vi "OAT Torsional Vibration (Analog Tacho) (Even-Angle) (N Ch - 1 Setting).vi"(0 "analog tacho signals":waveform(dbl)[](array[waveform]), 1 "threshold (auto)":dbl=inf, 2 "pulse/revolution (1)":i32=1 min=1, 3 "hysteresis (0)":dbl format="%.2g", 4 "torsional vibration units":enum16{"RPM", "deg/s", "rad/s"}(ring), 5 "error in (no error)":errorcluster, 6 "missing pulses? (no:F)":bool, 7 "pulse width (2)":i32=2 min=0, 8 "reset? (F)":bool, 9 "slope (Rising)":u16(ring) items=["Rising", "Falling"]) -> (14 "even-angle torsional vibration signals":cluster{"r0":dbl, "dr":dbl, "Y":dbl[]}[](array[cluster]) {"r0" format="%.2p"; "dr" format="%.2p"; "Y" format="%.2f"}, 15 "even-angle channel info":T3[](array[typedef]) {"channel info"."pregain" format="%.2f"; "channel info"."weighting filter" items=["Linear", "A-weighting", "B-weighting", "C-weighting", "ITU-R 468-4", "Dolby", "CCITT", "C-message", "Wb", "Wc", "Wd", "We", "Wf", "Wh", "Wj", "Wk", "Wm", "AES17 20 kHz lowpass", "AES17 40 kHz lowpass", "AES17 20 kHz highpass", "AES17 40 kHz highpass"]; "channel info"."dB reference" format="%^.1e"; "channel info"."engineering units" items=["custom..."=0, "V"=1, "A"=21, "C"=30, "pC"=31, "s"=32, "-"=29, "Pa"=2, "N"=20, "g"=3, "m/s^2"=4, "m/s"=5, "m"=6, "mm/s"=12, "mm"=13, "micron/s"=14, "micron"=15, "in/s^2"=7, "in/s"=8, "in"=9, "mil/s"=10, "mil"=11, "rad/s^2"=16, "rad/s"=17, "rad"=18, "deg/s^2"=26, "deg/s"=27, "deg"=28, "RPM"=22, "cycle/s^2"=23, "Hz"=24, "cycle"=25, "strain"=19]; "channel info"."sensor sensitivity" format="%#_5f"}, 16 "speed profiles":T2[](array[typedef]) {"speed [RPM]" format="%.2f"; "time [s]" format="%.2f"}, 17 "position info":T1[](array[typedef]), 18 "unit labels":string[](array[string]), 19 "error out":errorcluster)   [LabVIEW 2017, in "SoundVib_Torsional.lvlib"]
doc: "Calculates torsional vibration signals from analog tachometer signals. This VI can return torsional vibration signals as either waveform signals or even-angle signals. Wire data to the <B>analog tacho signal</B> input to determine the polymorphic instance to use or manually select the instance."
uses:
  <vilib>/addons/Sound and Vibration/Order Analysis/Torsional Vibration/SoundVib_Torsional.lvlib
  <vilib>/addons/_NISVFA/_Shared subVIs/Controls/svc_Resampled Channel Info.ctl
  <vilib>/addons/_NISVFA/_Shared subVIs/Controls/svc_Channel Info.ctl
  <vilib>/addons/_NISVFA/_Shared subVIs/Controls/svc_Engineering Units Text Ring.ctl
  <vilib>/addons/_NISVFA/_Shared subVIs/Controls/svc_Weighting Filter Text Ring.ctl
  <vilib>/addons/Sound and Vibration/Order Analysis/Tach Process/SubVIs/speed profile.ctl
  <vilib>/addons/Sound and Vibration/Order Analysis/Misc/OAT Position Info.ctl
  <vilib>/addons/_NISVFA/_Shared subVIs/Common/svc_Check for Waveform Parameter Continuity (no state).vi
  <vilib>/addons/_NISVFA/_Shared subVIs/Common/svc_Get SV Channel Info.vi
  <vilib>/addons/_NISVFA/_Shared subVIs/Common/svc_Engineering Units to Unit Label.vi
  <vilib>/addons/_NISVFA/_Shared subVIs/Common/svc_Unit Label to Engineering Units.vi
  <vilib>/addons/Sound and Vibration/Order Analysis/Tach Process/SoundVib_TachProcess.lvlib
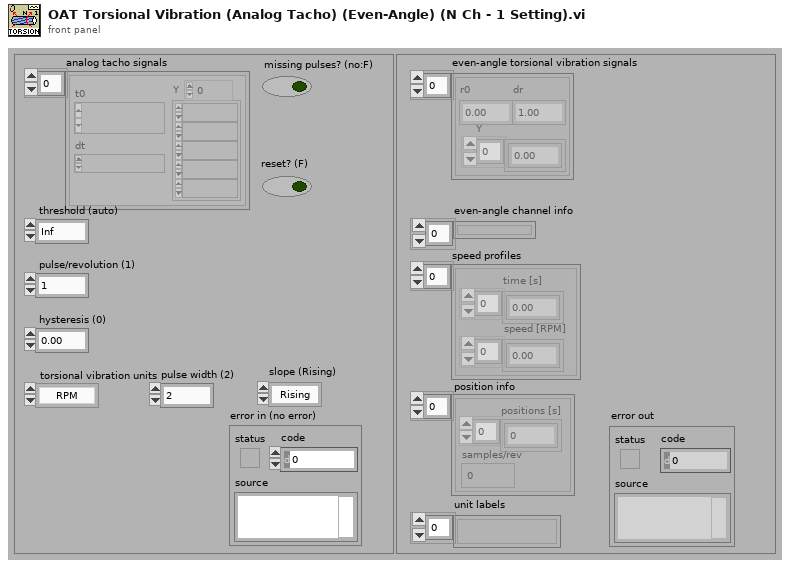
[diagram p1: front panel]
types:
  T1 = typedef "OAT Position Info.ctl" = cluster{"positions [s]":dbl[], "samples/rev":dbl}
  T2 = typedef "SoundVib_TachProcess.lvlib/speed profile.ctl" = cluster{"time [s]":dbl[], "speed [RPM]":dbl[]}
  T3 = typedef "svc_Resampled Channel Info.ctl" = cluster{"channel name":string, "description":string, " channel info":T4}
  T4 = typedef "svc_Channel Info.ctl" = cluster{"sensor sensitivity":dbl, "engineering units":T5, "dB reference":dbl, "custom label":string, "weighting filter":T6, "pregain":dbl}
  T5 = typedef "svc_Engineering Units Text Ring.ctl" = u16
  T6 = typedef "svc_Weighting Filter Text Ring.ctl" = u16
  T7 = cluster{"dt equal":bool, "array length equal":bool, "number channels change":bool}
  T8 = cluster{"dt":bool, "t0 continuity":bool, "array length":bool, "channel info":bool, "name":bool}
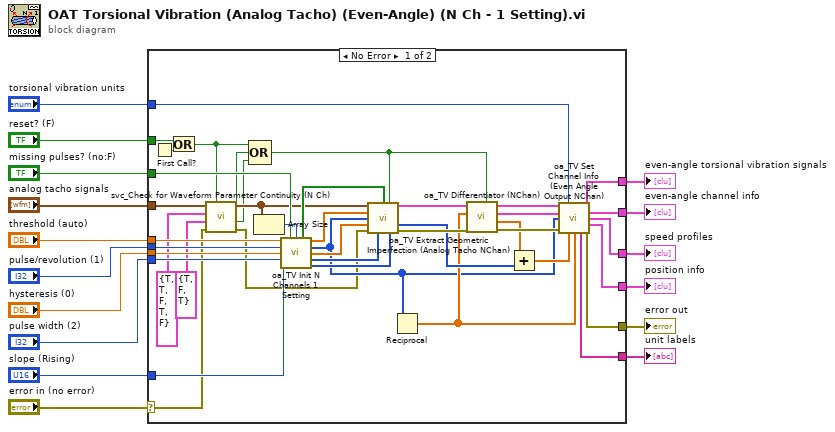
[diagram p0: block diagram]
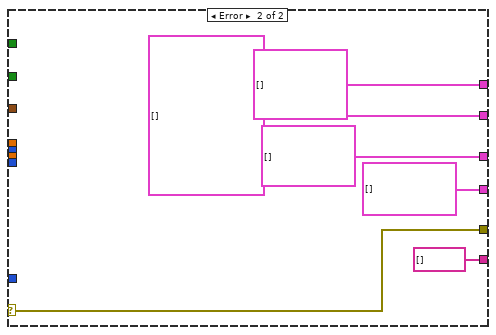
[diagram p2: hidden frame]
diagram:
  n1 = case shown="No Error" "error in (no error)" {
    selector: "error in (no error)" -> [w24 w63]
    tunnel: [w46 w63] -> w16
    tunnel: "reset? (F)" -> [w55 _]
    tunnel: "analog tacho signals" -> [w52 _]
    tunnel: [w42 cluster{"r0":dbl, "dr":dbl, "Y":dbl[]}[] []] -> w11
    tunnel: "torsional vibration units" -> [w40 _]
    tunnel: [w41 T3[] [] ("even-angle channel info")] -> w13
    tunnel: [w38 string[] [] ("unit labels")] -> w9
    tunnel: "threshold (auto)" -> [w36 _]
    tunnel: "pulse/revolution (1)" -> [w35 _]
    tunnel: "hysteresis (0)" -> [w34 _]
    tunnel: "pulse width (2)" -> [w33 _]
    tunnel: "slope (Rising)" -> [w32 _]
    tunnel: "missing pulses? (no:F)" -> [w31 _]
    tunnel: [w28 T2[] [] ("speed profiles")] -> w2
    tunnel: [w27 T1[] [] ("position info")] -> w1
    frame No Error {
      n2 = First Call?() -> (First Call?: T/F=w56:bool)
      n3 = Or(x=w55, y=w56) -> (x .or. y?=w22:bool)
      n4 = call <vilib>:"svc_Check for Waveform Parameter Continuity (N Ch).vi"("restart averaging (F)"=w22, "error in (no error)"=w24, "checks for multichannel parameters"=T7 {"dt equal"=TRUE, "array length equal"=FALSE, "number channels change"=TRUE}, "checks for channel parameter change"=T8 {"dt"=TRUE, "t0 continuity"=TRUE, "array length"=FALSE, "channel info"=TRUE, "name"=FALSE}, "scaled signal(s)"=w52) -> ("error out"=w23:errorcluster, "multichannel parameter changed"=w19:bool, "waveform parameter changed"=w20:bool, "dup scaled signal(s)"=w25:waveform(dbl)[])  [unwired: 3 out]
      n5 = Compound Arithmetic op=OR(w22, w20, w19) -> (w21:bool)
      n6 = Array Size(array=w25) -> (size(s)=w51:i32)
      n7 = call <vilib>:"oa_TV Init N Channels 1 Setting.vi"("threshold (auto)"=w36, "missing pulses? (no:F)"=w31, "channel number"=w51, "pulse/revolution (1)"=w35, "hysteresis (0)"=w34, "pulse width (2)"=w33, "slope (Rising)"=w32) -> ("missing pulses? out"=w50:bool[], "threshold out"=w49:dbl[], "pulse/revolution out"=w29:i32[], "hysteresis"=w37:dbl[], "pulse width out"=w39:i32[], "slope out"=w48:u16[])  [unwired: 2 in, 1 out]
      n8 = call <vilib>:"oa_TV Extract Geometric Imperfection (Analog Tacho NChan).vi"("analog tacho signal"=w25, "missing pulses? (no:F)"=w50, "reset? (F)"=w21, "threshold (auto)"=w49, "pulse/revolution"=w29, "hysteresis(0)"=w37, "error in (no error)"=w23, "pulse width (2)"=w39, "slope (Rising)"=w48) -> ("pulse positions"=w53:cluster{dbl[]}[], "revulotion index"=w54:i32[], "error out"=w57:errorcluster)  [unwired: 3 in, 1 out]
      n9 = Reciprocal(x=w29) -> (1/x=w45:dbl[])
      n10 = call <vilib>:"oa_TV Differentiator (NChan).vi"("reset? (False)"=w21, "error in (no error)"=w57, "delta X"=w45, "Y[n]"=w53) -> ("error out"=w47:errorcluster, "Delay"=w26:dbl[], "X[n]"=w30:cluster{dbl[]}[], "dY[n]/dX[n]"=w43:cluster{dbl[]}[])  [unwired: 4 in]
      n11 = Add(x=w26, y=w54) -> (x+y=w44:dbl[])
      n12 = call <vilib>:"oa_TV Set Channel Info (Even Angle Output NChan).vi"("seconds/revolution"=w43, "torisional vibration unit (RPM)"=w40, "pulse positions"=w30, "pulse/revolution (1)"=w29, "error in (no error)"=w47, "r0"=w44, "dr"=w45) -> ("even-angle torsional vibration"=w42:cluster{"r0":dbl, "dr":dbl, "Y":dbl[]}[], "even-angle channel info"=w41:T3[], "speed profiles"=w28:T2[], "position info"=w27:T1[], "unit labels"=w38:string[], "error out"=w46:errorcluster)  [unwired: 3 in]
    }
    frame Error {
    }
  }
  "error out" <- w16
  "even-angle channel info" <- w13
  "even-angle torsional vibration signals" <- w11
  "unit labels" <- w9
  "speed profiles" <- w2
  "position info" <- w1
